vi "test Source Separated.vi"(8 "error in (no error)":errorcluster, 11 "TestCase in":refnum<class "SLSC EDS Unit Tests.lvclass">) -> (0 "error out":errorcluster, 3 "TestCase out":refnum<class "SLSC EDS Unit Tests.lvclass">)   [LabVIEW 2015, in "SLSC EDS Unit Tests.lvclass"]
uses:
  SLSC EDS Unit Tests.lvclass
  <vilib>/addons/_JKI Toolkits/VI Tester/TestCase.llb/TestCase.lvclass
  niveristand-custom-device-testing-tools/VeriStandTestUtilities/VeriStandTestUtilities.lvlib
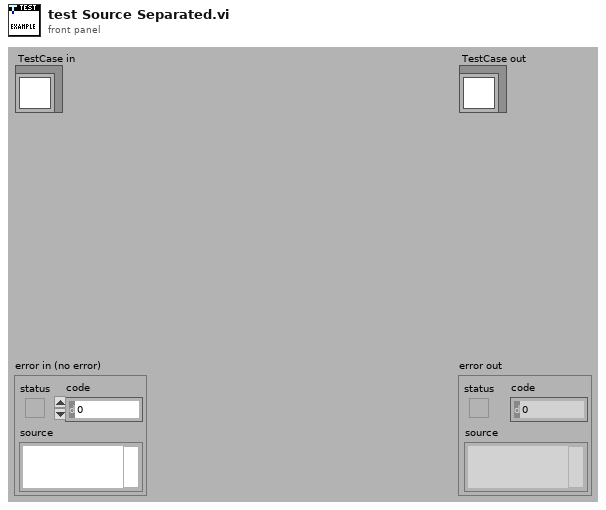
[diagram p1: front panel]
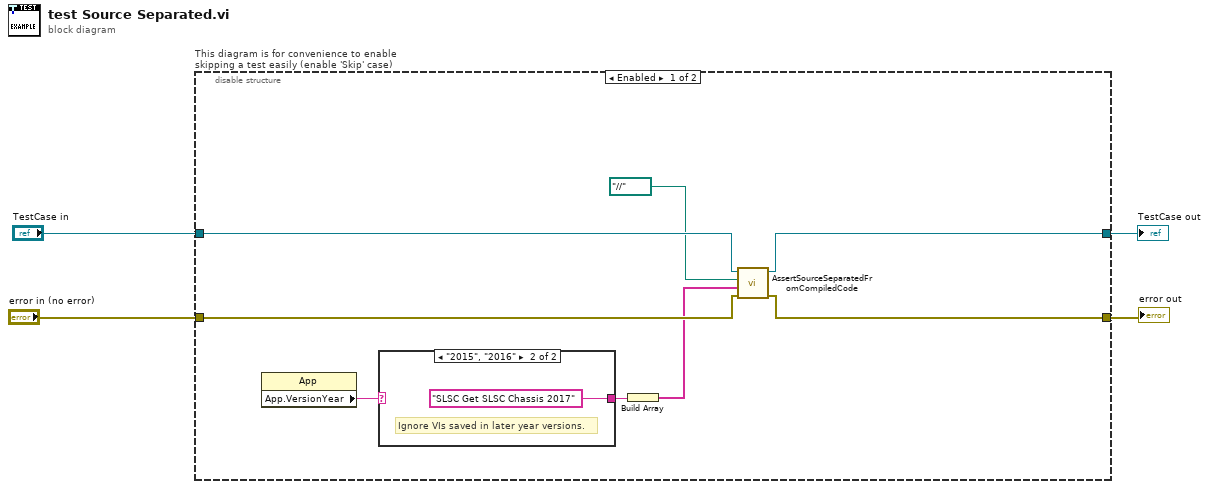
[diagram p0: block diagram]
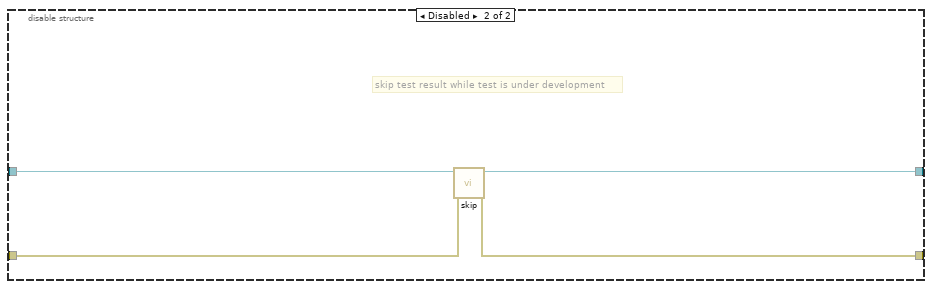
[diagram p3: hidden frame]
diagram:
  n1 = disable-structure "This diagram is for convenience to enable skipping a test easily (enable 'Skip' case)" shown="Enabled" {
    disable-tunnel: "TestCase in" -> [w10 w17]
    disable-tunnel: [w9 w15] -> w1
    disable-tunnel: [w11 w16] -> w3
    disable-tunnel: "error in (no error)" -> [w12 w14]
    frame Enabled {
      n2 = property class="App"() -> ("App.VersionYear"=w7:string)  [unwired: 2 in, 2 out]
      n3 = case shown="\"2015\", \"2016\"" w7 {
        tunnel: [_ "SLSC Get SLSC Chassis 2017"] -> w6
        frame Default {
        }
        frame "2015", "2016" {
          # "Ignore VIs saved in later year versions."
        }
      }
      n4 = Build Array(w6) -> (w5:string[])
      n5 = call "AssertSourceSeparatedFromCompiledCode.vi"("error in (no error)"=w12, "folders to exclude"=w5, "search path"=path "../../..", "TestCase in"=w10) -> ("error out"=w11:errorcluster, "TestCase out"=w9:refnum<class "SLSC EDS Unit Tests.lvclass">)  [unwired: 6 in]
    }
    frame Disabled {
      # "skip test result while test is under development"
      n6 = call <vilib>:"skip.vi"("error in (no error)"=w14, "TestCase in"=w17) -> ("error out"=w16:errorcluster, "TestCase out"=w15:refnum<class "SLSC EDS Unit Tests.lvclass">)  [unwired: 8 in]
    }
  }
  "error out" <- w3
  "TestCase out" <- w1
